vi "End Array.vi"   [LabVIEW 2017, in "LabPack.lvlib" / "Writer.lvclass"]
uses:
  Writer.lvclass
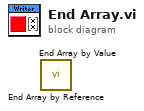
[diagram p0: block diagram]
diagram:
  n1 = call "End Array by Reference.vi"() -> ()  [unwired: 10 in, 2 out]
  n2 = call "End Array by Value.vi"() -> ()  [unwired: 10 in, 2 out]
